vi "Next State.vi"(11 "Fan ON":bool) -> (3 "s? t:f":T1)   [LabVIEW 2021]
uses:
  Type defs/Fan STates.ctl
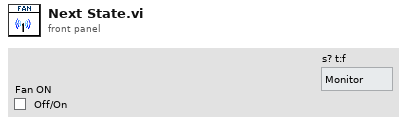
[diagram p1: front panel]
types:
  T1 = typedef "Fan STates.ctl" = enum16{"Monitor", "Fan On"}
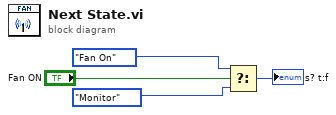
[diagram p0: block diagram]
diagram:
  n1 = Select(t=Fan_STates."Fan On", s="Fan ON", f=Fan_STates."Monitor") -> (s? t:f=→"s? t:f":T1)
